vi "regGenReadUserEvent.vi"(8 "error in (no error)":errorcluster, 11 "TcpServerBase in":refnum<class "TcpServerBase.lvclass">) -> (0 "error out":errorcluster, 3 "TcpServerBase out":refnum<class "TcpServerBase.lvclass">)   [LabVIEW 2018, in "TcpServerBase.lvclass"]
doc: "Register the GenRead user event."
uses:
  TcpServerBase.lvclass
  typedef/connStatusCluster.ctl
  TcpServerBase.lvclass/TcpServerBase.ctl
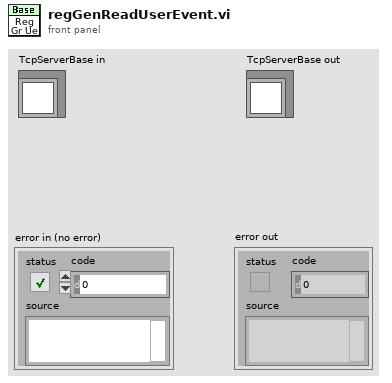
[diagram p1: front panel]
types:
  T1 = typedef "TcpServerBase.lvclass/connStatusCluster.ctl" = cluster{"areClientsConnected":enum16{"unchanged", "connected", "unconnected"}, "connStatusMsg":string}
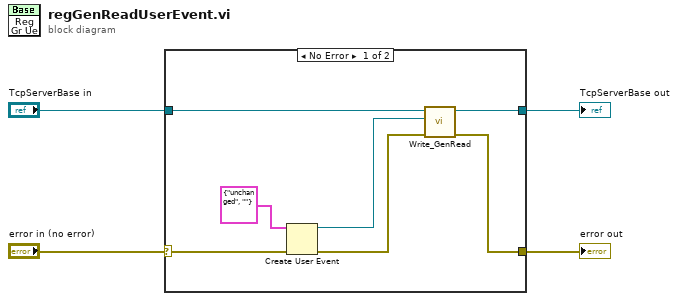
[diagram p0: block diagram]
diagram:
  n1 = case shown="No Error" "error in (no error)" {
    selector: "error in (no error)" -> [w9 w12]
    tunnel: "TcpServerBase in" -> [w11 w13]
    tunnel: [w10 w13] -> w3
    tunnel: [w6 w12] -> w1
    frame No Error {
      n2 = Create User Event(user event datatype=T1 {"areClientsConnected"=enum."unchanged", "connStatusMsg"=""} ("connStatusCluster"), error in=w9) -> (user event=w8:refnum<user-event>, error out=w7:errorcluster)
      n3 = call "Write_GenRead.vi"("error in (no error)"=w7, "GenRead"=w8, "TcpServerBase in"=w11) -> ("error out"=w6:errorcluster, "TcpServerBase out"=w10:refnum<class "TcpServerBase.lvclass">)  [unwired: 7 in]
    }
    frame Error {
    }
  }
  "TcpServerBase out" <- w3
  "error out" <- w1
